vi "Add Folder Path to Tree.vi"(8 "error in (no error)":errorcluster, 9 "All Folder Tags":string[](array[string]), 10 "Folder Path":path, 11 "TreeControl in":refnum<vi>) -> (0 "error out":errorcluster, 1 "All Folder Tags Out":string[](array[string]), 2 "Folder Item Tag":string)   [LabVIEW 2013, in "LVTM.lvlib"]
uses:
  LVTM.lvlib
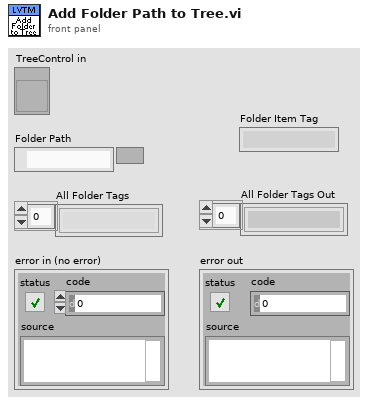
[diagram p1: front panel]
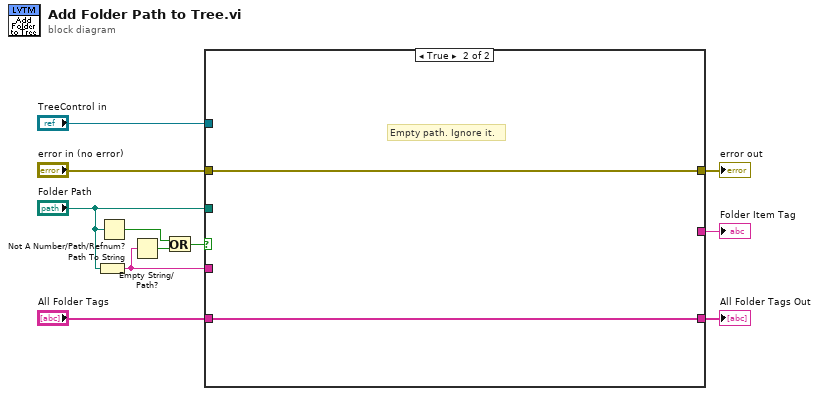
[diagram p0: block diagram]
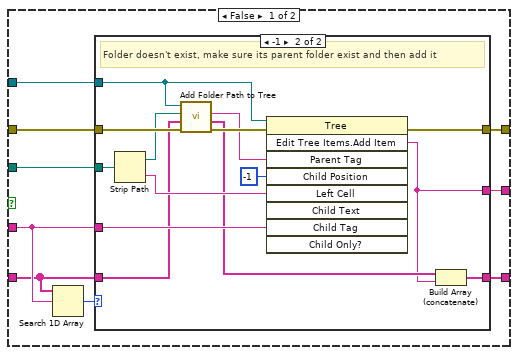
[diagram p2: hidden frame]
diagram:
  n1 = Path To String(path="Folder Path") -> (string=w5:string)
  n2 = Not A Number/Path/Refnum?(number/path/refnum="Folder Path") -> (NaN/Path/Refnum?=w1:bool)
  n3 = Empty String/Path?(string/path=w5) -> (empty?=w4:bool)
  n4 = Or(x=w1, y=w4) -> (x .or. y?=w2:bool)
  n5 = case shown="True" w2 {
    tunnel: [w20 w38] -> w11
    tunnel: [w19 w39] -> w10
    tunnel: "error in (no error)" -> [w18 w39]
    tunnel: w5 -> [w17 _]
    tunnel: "Folder Path" -> [w15 _]
    tunnel: "All Folder Tags" -> [w14 w38]
    tunnel: "TreeControl in" -> [w13 _]
    tunnel: [w12 _] -> w6
    frame False {
      n6 = Search 1D Array(1D array=w14, element=w17) -> (index of element=w16:i32)  [unwired: 1 in]
      n7 = case shown="-1" w16 {
        tunnel: w13 -> [_ w28]
        tunnel: w14 -> [w23 w30]
        tunnel: w17 -> [w21 w37]
        tunnel: w15 -> [_ w27]
        tunnel: [w23 w34] -> w20
        tunnel: w18 -> [w22 w32]
        tunnel: [w22 w33] -> w19
        tunnel: [w21 w25] -> w12
        frame 0, Default {
          # "Path already exists"
        }
        frame -1 {
          # "Folder doesn't exist, make sure its parent folder exist and then add it"
          n8 = Strip Path(path=w27) -> (stripped path=w26:path, name=w36:string)
          n9 = call "Add Folder Path to Tree.vi"("error in (no error)"=w32, "All Folder Tags"=w30, "Folder Path"=w26, "TreeControl in"=w28) -> ("error out"=w31:errorcluster, "All Folder Tags Out"=w29:string[], "Folder Item Tag"=w24:string)  [unwired: 5 in]
          n10 = invoke on="Invoke Node" class="Tree" method="Edit Tree Items.Add Item"(reference=w28, error in=w31, "Parent Tag"=w24, "Child Position"=-1, "Left Cell"=w36, "Child Tag"=w37) -> (error out=w33:errorcluster, "Edit Tree Items:Add Item"=w25:string)  [unwired: 3 in, 7 out]
          n11 = Build Array (concatenate)(w29, w25) -> (w34:string[])
        }
      }
    }
    frame True {
      # "Empty path. Ignore it."
    }
  }
  "All Folder Tags Out" <- w11
  "error out" <- w10
  "Folder Item Tag" <- w6
